vi "Example Threshold - VoltageReached Callback.vi"(4 "VoltageReached":refnum<user-event>, 5 "Event Data":T1, 6 "Control Ref":refnum<k24>, 7 "Event Common Data":T2) -> ()   [LabVIEW 2013]
uses:
  C:/tf/play/labview/Tinkerforge.dll
  Tinkerforge.dll
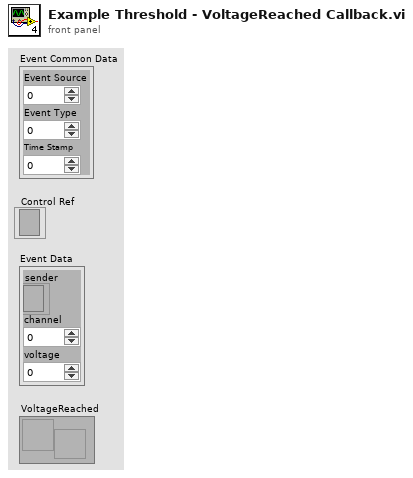
[diagram p1: front panel]
types:
  T1 = cluster{"sender":refnum<k24>, "channel":u8, "voltage":i32}
  T2 = cluster{"Event Source":i32, "Event Type":u32, "Time Stamp":u32}
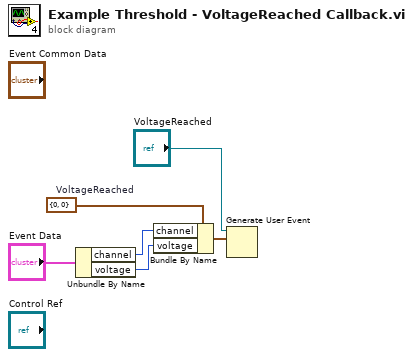
[diagram p0: block diagram]
diagram:
  w6 = cluster{"channel":u8, "voltage":i32} {"channel"=0, "voltage"=0}  # VoltageReached
  n1 = Unbundle By Name("Event Data") -> ("channel"=w3:u8, "voltage"=w2:i32)
  n2 = Bundle By Name(cluster=w6, "channel"=w3, "voltage"=w2) -> (w5:cluster{"channel":u8, "voltage":i32})
  n3 = Generate User Event(user event="VoltageReached", event data cluster=w5) -> ()  [unwired: 2 in, 2 out]
